vi "ryTimerEx Queue Ignore If Exists.vi"() -> ()   [LabVIEW 2020]
uses:
  3122cb75-6530-49f8-9864-937ee694b227.vi
  Lib/ryTimer.lvclass
panel:
  in  "Exit":bool
  out "Elements in Queue":string[](array[string])
  out "Error":errorcluster
  # "Should only have\none \"READ\" element\nenqueued at a time"
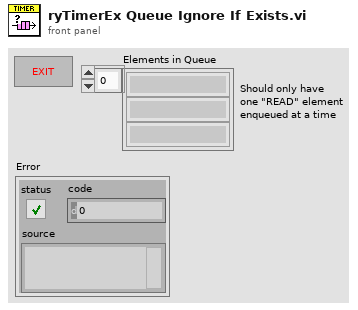
[diagram p1: front panel]
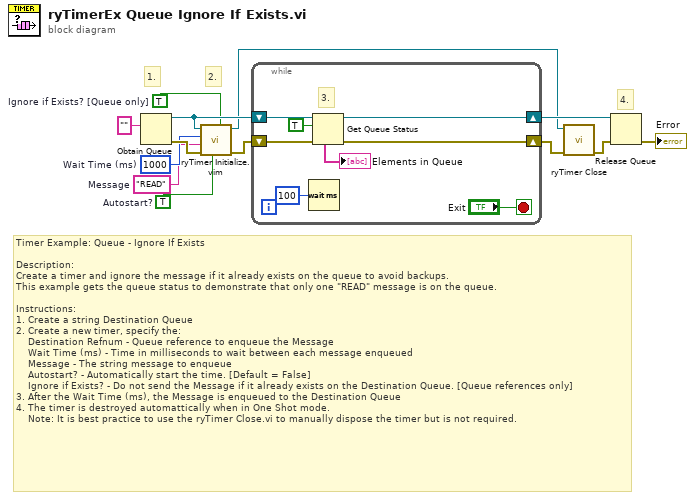
[diagram p0: block diagram]
diagram:
  w4 = TRUE  # Ignore if Exists? [Queue only]
  w9 = TRUE  # Autostart?
  w10 = "READ"  # Message
  w11 = u32 1000  # Wait Time (ms)
  # "Timer Example: Queue - Ignore If Exists\n\nDescription:\nCreate a timer and ignore the message if it already exists on the queue to avoid backups.\nThis example gets the queue status to demonstrate that only one \"READ\" message is on the queue.\n\nInstructions:\n1. Create a string Destination Queue\n2. Create a new timer, specify the:\n    Destination Refnum - Queue reference to enqueue the Message\n    Wait Time (ms) - Time in milliseconds to wait between each message enqueued\n    Message - The string message to enqueue\n    Autostart? - Automatically start the time. [Default = False]\n    Ignore if Exists? - Do not send the Message if it already exists on the Destination Queue. [Queue references only]\n3. After the Wait Time (ms), the Message is enqueued to the Destination Queue\n4. The timer is destroyed automattically when in One Shot mode.\n    Note: It is best practice to use the ryTimer Close.vi to manually dispose the timer but is not required."
  # "4."
  # "2."
  # "1."
  n1 = Obtain Queue(element data type="") -> (queue out=w8:refnum<queue>, error out=w12:errorcluster)  [unwired: 4 in, 1 out]
  n2 = call "ryTimer Initialize.vim"("Ignore if Exists? (F) [Queue only]"=w4, "Autostart? (F)"=w9, "error in (no error)"=w12, "Message"=w10, "Wait Time (ms)"=w11, "Destination Refnum [Q,UE,Any]"=w8) -> ("error out"=w5:errorcluster, "Timer out"=w1:refnum<class "ryTimer.lvclass">)  [unwired: 4 in]
  n3 = while {
    shift-right: [w20] -> w6
    shift-left: w8 -> [w21]
    shift-right: [w18] -> w3
    shift-left: w5 -> [w19]
    stop <- "Exit" stop-if-true
    # "3."
    n4 = Wait (ms)(milliseconds to wait=u32 100) -> ()  [unwired: 1 out]
    n5 = Get Queue Status(queue=w21, return elements? (F)=TRUE, error in (no error)=w19) -> (queue out=w20:refnum<queue>, error out=w18:errorcluster, elements=→"Elements in Queue":string[])  [unwired: 5 out]
  }
  n6 = call "ryTimer Close.vi"("error in (no error)"=w3, "Timer in"=w1) -> ("error out"=w2:errorcluster)  [unwired: 9 in]
  n7 = Release Queue(queue=w6, error in (no error)=w2) -> (error out=→"Error":errorcluster)  [unwired: 1 in, 2 out]
